vi "GetOldData.vi"(5 "LogPath":path) -> (0 "log":string, 1 "clients":string, 2 "server":string)   [LabVIEW 2018]
doc: "Deletes old data from logs"
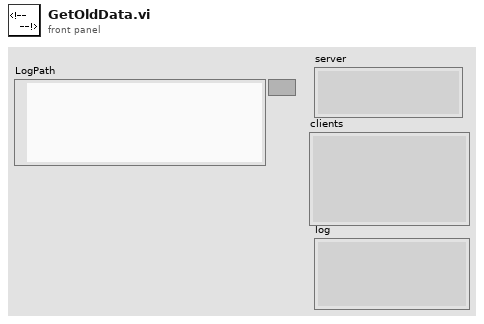
[diagram p1: front panel]
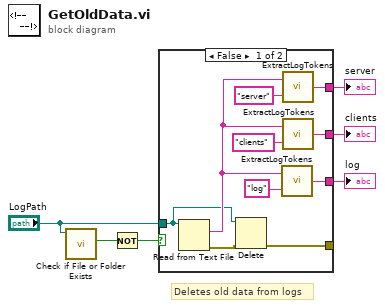
[diagram p0: block diagram]
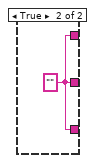
[diagram p2: hidden frame]
diagram:
  # "Deletes old data from logs"
  n1 = call <vilib>:"Check if File or Folder Exists.vi"("path"="LogPath") -> ("file or folder exists?"=w2:bool)  [unwired: 8 in, 2 out]
  n2 = Not(x=w2) -> (.not. x?=w3:bool)
  n3 = case shown="False" w3 {
    tunnel: "LogPath" -> [w9 _]
    tunnel: [w15 w17] -> w6
    tunnel: [w13 w17] -> w1
    tunnel: [w10 w17] -> w5
    tunnel: [w8 _] -> _
    frame False {
      n4 = Read from Text File(file (use dialog)=w9) -> (text=w11:string, error out=w7:errorcluster)  [unwired: 3 in, 2 out]
      n5 = Delete(path (use dialog)=w9, error in=w7) -> (error out=w8:errorcluster)  [unwired: 3 in, 2 out]
      n6 = call <userlib>:"ExtractLogTokens.vi"("HTML"=w11, "section"="log" ("string")) -> ("tagged text"=w15:string)  [unwired: 2 out]
      n7 = call <userlib>:"ExtractLogTokens.vi"("HTML"=w11, "section"="server" ("string")) -> ("tagged text"=w13:string)  [unwired: 2 out]
      n8 = call <userlib>:"ExtractLogTokens.vi"("HTML"=w11, "section"="clients" ("string")) -> ("tagged text"=w10:string)  [unwired: 2 out]
    }
    frame True {
      w17 = ""
    }
  }
  "log" <- w6
  "clients" <- w5
  "server" <- w1
